vi "MoveSubVI.vi"(1 "M1":bool, 2 "M0":bool, 4 "error in (no error)":errorcluster, 5 "Direction":bool, 6 "Number of Steps":u32, 7 "LINX Resource":T1) -> (0 "error out":errorcluster, 3 "LINX Resource 2":T1)   [LabVIEW 2021]
uses:
  <vilib>/MakerHub/LINX/Private/Type Defs/LINX Ref.ctl
  <vilib>/MakerHub/LINX/Private/Type Defs/Platform.ctl
  <vilib>/MakerHub/LINX/Private/Type Defs/Interface.ctl
  <vilib>/MakerHub/LINX/Private/Device/Type Defs/LINX Device Config.ctl
  <vilib>/MakerHub/LINX/Private/Device/Type Defs/TCP Config.ctl
  <vilib>/MakerHub/LINX/Private/Device/Type Defs/Channels.ctl
  <vilib>/MakerHub/LINX/Public/Peripherals/Digital/Digital Write 1 Chan.vi
  <vilib>/MakerHub/LINX/Public/Peripherals/Digital/Digital Write N Chans.vi
  <vilib>/MakerHub/LINX/Private/Local IO/LinxDigitalWrite.vi
  <vilib>/MakerHub/LINX/Public/Utilities/Check Channel.vi
  <vilib>/MakerHub/LINX/Private/Utilties/Generate Error.vi
  <vilib>/MakerHub/LINX/LMH-LINX.lvlib
  <vilib>/MakerHub/LINX/Private/Device/Device.lvlib
panel:
  out "PIN Step":u8=11
  out "PIN Dir":u8=12
  out "PIN M1":u8=9
  out "PIN M0":u8=8
  # "Function & M0 & M1\n ----------------------\nFull  Step:       0         0\n1/2   Step:       1         0\n1/8   Step:       0         1\n1/16 Step:       1         1"
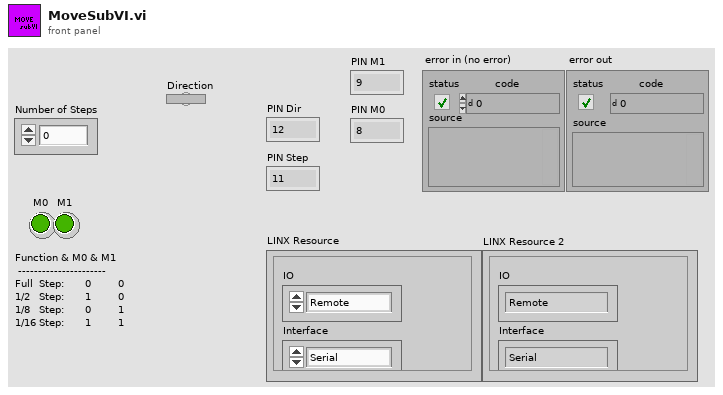
[diagram p1: front panel]
types:
  T1 = typedef "LMH-LINX.lvlib/LINX Ref.ctl" = cluster{"IO":T2, "Interface":T3, "LINX Device Config":T4}
  T2 = typedef "LMH-LINX.lvlib/Platform.ctl" = enum16{"Remote", "Local"}
  T3 = typedef "LMH-LINX.lvlib/Interface.ctl" = enum16{"Serial", "TCP"}
  T4 = typedef "LMH-LINX.lvlib/Device.lvlib/LINX Device Config.ctl" = cluster{"Interface":T3, "COM Port":refnum<visa-resource-name>, "TCP Configuration":T5, "Device Family":u8, "Device ID":u8, "Device Name":string, "TCP Ref":refnum<k5>, "Channels":T6}
  T5 = typedef "LMH-LINX.lvlib/Device.lvlib/TCP Config.ctl" = cluster{"IP Address":string, "Port":u16}
  T6 = typedef "LMH-LINX.lvlib/Channels.ctl" = cluster{"DI":u8[], "DO":u8[], "AI":u8[], "AO":u8[], "PWM":u8[], "QE":u8[], "UART":u8[], "I2C 2":u8[], "SPI":u8[], "CAN":u8[], "Servo":u8[], "AI Ref (V)":dbl, "AI Resolution (Bits)":u8, "AO Ref (V)":dbl, "AO Resolution (Bits)":u8}
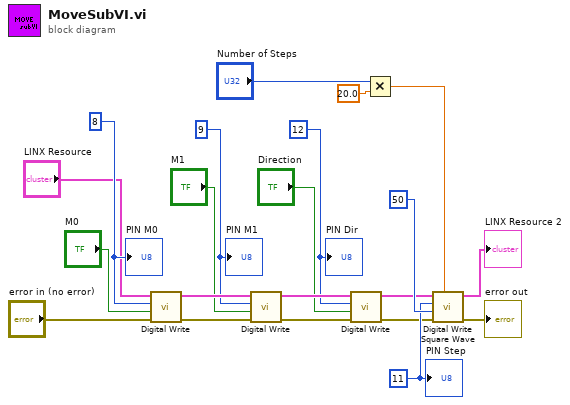
[diagram p0: block diagram]
diagram:
  w13 = u8 12 ("DO Channel")
  w15 = u8 9 ("DO Channel")
  w17 = u8 8 ("DO Channel")
  w18 = u8 11 ("Channel")
  n1 = call-poly <vilib>:"Digital Write.vi"("Error In"="error in (no error)", "Output Value"="M0", "DO Channel"=w17, "LINX Resource"="LINX Resource") -> ("Error Out"=w12:errorcluster, "LINX Resource"=w16:T1)  [unwired: 6 in]
  n2 = call-poly <vilib>:"Digital Write.vi"("Error In"=w12, "Output Value"="M1", "DO Channel"=w15, "LINX Resource"=w16) -> ("Error Out"=w11:errorcluster, "LINX Resource"=w14:T1)  [unwired: 6 in]
  n3 = call-poly <vilib>:"Digital Write.vi"("Error In"=w11, "Output Value"="Direction", "DO Channel"=w13, "LINX Resource"=w14) -> ("Error Out"=w10:errorcluster, "LINX Resource"=w9:T1)  [unwired: 6 in]
  n4 = Multiply(x="Number of Steps", y=20.0) -> (x*y=w20:dbl)
  n5 = call <vilib>:"Digital Write Square Wave.vi"("Duration (ms)"=w20, "Error In"=w10, "Frequency (Hz)"=u32 50, "Channel"=w18, "LINX Resource"=w9) -> ("Error Out"=→"error out":errorcluster, "LINX Resource"=→"LINX Resource 2":T1)  [unwired: 5 in]
  "PIN M0" <- w17
  "PIN M1" <- w15
  "PIN Dir" <- w13
  "PIN Step" <- w18
